vi "ERIO WIN Process Notifications.vi"(6 "Supervisory Variables In":T1={"Alarm Threshold"=0.0, "Shutdown"=FALSE, "Enable SNS Alarm"=FALSE, "Enable SNS Stage Notification"=FALSE, "Enable SQS Notification"=FALSE, "Enable S3 TDMS Signal Capture"=FALSE, "Enable SystemLink Signal Capture"=FALSE, "Capture Signal"=FALSE, "Server Update"=FALSE, "AWS Access Key"="AKIAINLDO2Y2PDFEWDOQ", "AWS Secret Key"="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", "Phone Number"="+15037066913", "Region"=enum."us-west-2", "AWS SQS Queue"="+15037066913", "AWS S3 Bucket"="+15037066913"}, 7 "WIN Variables In":T3, 8 "error in (no error)":errorcluster, 9 "AWS Variables In":T5, 11 "EEISysLink.lvclass In":refnum<class "EEISysLink.lvclass">) -> (0 "error out":errorcluster, 1 "AWS Variables Out":T5, 3 "EEISysLink.lvclass Out":refnum<class "EEISysLink.lvclass">, 4 "Supervisory Variables Out":T1={"Alarm Threshold"=0.0, "Shutdown"=FALSE, "Enable SNS Alarm"=FALSE, "Enable SNS Stage Notification"=FALSE, "Enable SQS Notification"=FALSE, "Enable S3 TDMS Signal Capture"=FALSE, "Enable SystemLink Signal Capture"=FALSE, "Capture Signal"=FALSE, "Server Update"=FALSE, "AWS Access Key"="AKIAINLDO2Y2PDFEWDOQ", "AWS Secret Key"="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", "Phone Number"="+15037066913", "Region"=enum."us-west-2", "AWS SQS Queue"="+15037066913", "AWS S3 Bucket"="+15037066913"}, 5 "WIN Variables Out":T3)   [LabVIEW 2017]
doc: "Check for notifications from AWS SNS service and if found process/display them. \n\nJames Tillett P.E.\nEndeavor Engineering Inc.\nwww.endeavoreng.com"
uses:
  Class EEISysLink/EEISysLink.lvclass
  Controls/ERIO AWS Toolkit Variables.ctl
  <vilib>/AWS Toolkit/SQS/Queue/Queue.lvclass
  <vilib>/AWS Toolkit/SNS/Phone Number/Phone Number.lvclass
  <vilib>/AWS Toolkit/S3/Bucket/Bucket.lvclass
  Controls/ERIO Supervisory Variables.ctl
  <vilib>/AWS Toolkit/Core/HTTP Request/Region.ctl
  Controls/ERIO WIN State Variables.ctl
  Controls/ERIO Worker Variables.ctl
  <vilib>/AWS Toolkit/Core/HTTP Request/HTTP Request.lvclass
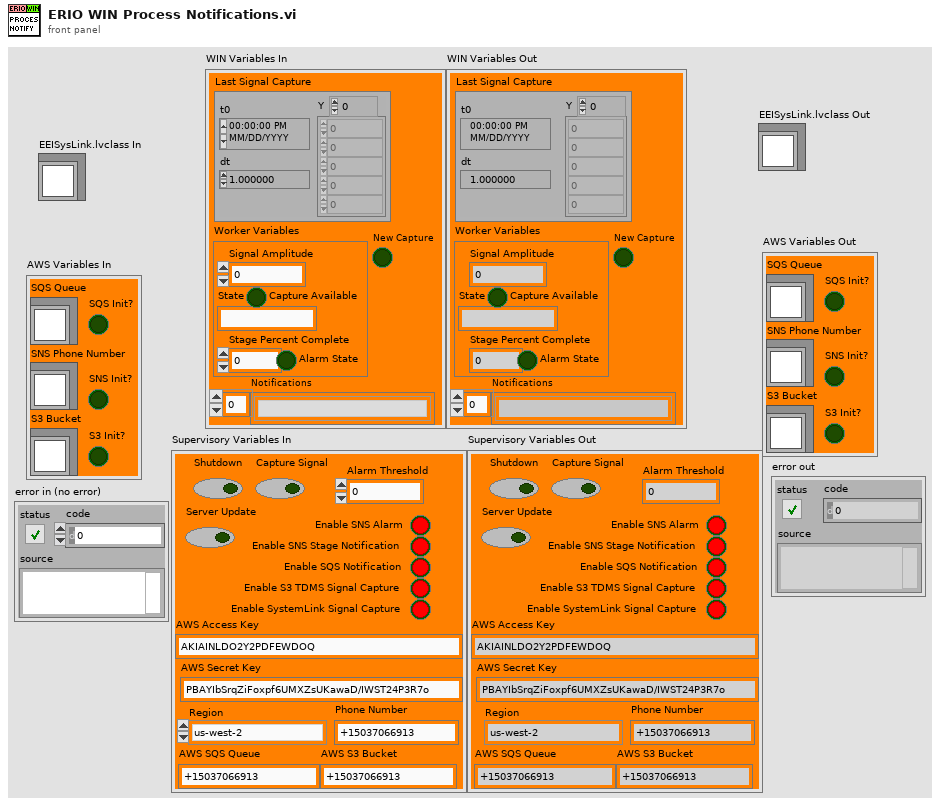
[diagram p1: front panel]
types:
  T1 = typedef "ERIO Supervisory Variables.ctl" = cluster{"Alarm Threshold":dbl, "Shutdown":bool, "Enable SNS Alarm":bool, "Enable SNS Stage Notification":bool, "Enable SQS Notification":bool, "Enable S3 TDMS Signal Capture":bool, "Enable SystemLink Signal Capture":bool, "Capture Signal":bool, "Server Update":bool, "AWS Access Key":string, "AWS Secret Key":string, "Phone Number":string, "Region":T2, "AWS SQS Queue":string, "AWS S3 Bucket":string}
  T2 = typedef "NI_AWS_Core.lvlib/HTTP Request.lvclass/Region.ctl" = enum16{"us-east-1", "us-east-2", "us-west-1", "us-west-2", "ap-northeast-1", "ap-northeast-2", "ap-southeast-1", "ap-southeast-2", "ca-central-1", "eu-central-1", "eu-west-1", "eu-west-2", "sa-east-1"}
  T3 = typedef "ERIO WIN State Variables.ctl" = cluster{"Worker Variables":T4, "Notifications":string[], "New Capture":bool, "Last Signal Capture":waveform(dbl)}
  T4 = typedef "ERIO Worker Variables.ctl" = cluster{"Signal Amplitude":dbl, "State":string, "Stage Percent Complete":dbl, "Alarm State":bool, "Capture Available":bool}
  T5 = typedef "ERIO AWS Toolkit Variables.ctl" = cluster{"SQS Queue":refnum<class "Queue.lvclass">, "SNS Phone Number":refnum<class "Phone Number.lvclass">, "S3 Bucket":refnum<class "Bucket.lvclass">, "SQS Init?":bool, "S3 Init?":bool, "SNS Init?":bool}
  T6 = typedef "NI_AWS_SQS.lvlib/Queue.lvclass/Message.ctl" = cluster{"Body":string, "MD5 of Body":string, "ID":string, "Receipt Handle":string, "Native Attributes":T7[], "Custom Attributes":T9[], "MD5 of Custom Attributes":string}
  T7 = typedef "NI_AWS_SQS.lvlib/Queue.lvclass/Message Attribute Value Pair.ctl" = cluster{"Attribute":T8, "Value":string}
  T8 = typedef "NI_AWS_SQS.lvlib/Queue.lvclass/Message Attribute.ctl" = enum16{"SenderId", "SentTimestamp", "ApproximateReceiveCount", "ApproximateFirstReceiveTimestamp"}
  T9 = typedef "NI_AWS_SQS.lvlib/Queue.lvclass/Custom Attribute.ctl" = cluster{"Name":string, "Type":T10, "Value":string}
  T10 = typedef "NI_AWS_SQS.lvlib/Queue.lvclass/Custom Attribute Type.ctl" = enum16{"String", "Number", "Binary"}
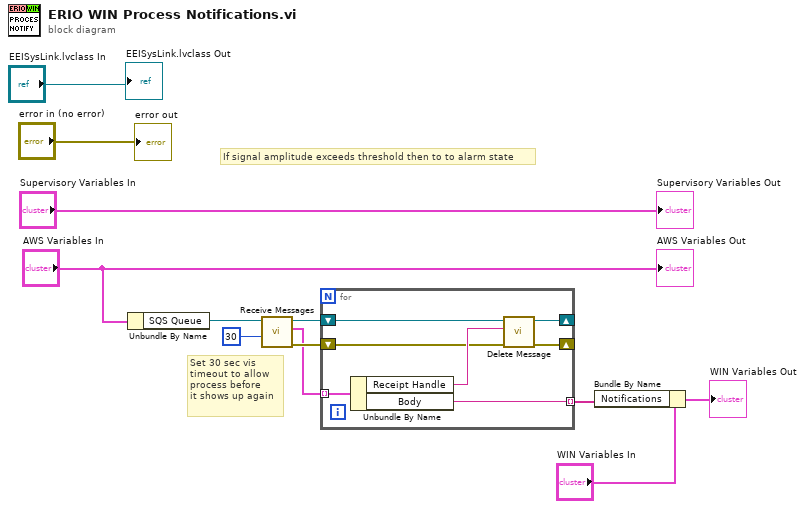
[diagram p0: block diagram]
diagram:
  # "Set 30 sec vis\ntimeout to allow\nprocess before\nit shows up again"
  # "If signal amplitude exceeds threshold then to to alarm state"
  n1 = Unbundle By Name("AWS Variables In") -> ("SQS Queue"=w4:refnum<class "Queue.lvclass">)
  n2 = call <vilib>:"Receive Messages.vi"("Visibility Timeout"=30, "SQS in"=w4) -> ("error out"=w10:errorcluster, "Messages"=w8:T6[], "SQS out"=w9:refnum<class "Queue.lvclass">)  [unwired: 7 in]
  n3 = for {
    tunnel: w8 -> [w19] mode=indexing
    shift-right: [w15] -> _
    shift-left: w9 -> [w18]
    shift-right: [w14] -> _
    shift-left: w10 -> [w16]
    tunnel: [w13] -> w3 mode=indexing
    n4 = Unbundle By Name(w19) -> ("Receipt Handle"=w17:string, "Body"=w13:string)
    n5 = call <vilib>:"Delete Message.vi"("error in (no error)"=w16, "Receipt Handle"=w17, "SQS in"=w18) -> ("error out"=w14:errorcluster, "SQS out"=w15:refnum<class "Queue.lvclass">)  [unwired: 7 in]
  }
  n6 = Bundle By Name(cluster="WIN Variables In", "Notifications"=w3) -> (→"WIN Variables Out":T3)
  "EEISysLink.lvclass Out" <- "EEISysLink.lvclass In"
  "error out" <- "error in (no error)"
  "AWS Variables Out" <- "AWS Variables In"
  "Supervisory Variables Out" <- "Supervisory Variables In"
